vi "DAQmx-AI.GetPrivateEvents.vi"(8 "error in (no error)":errorcluster, 11 "DAQmx-AI":refnum<class "DAQmx-AI.lvclass">) -> (0 "error out":errorcluster, 2 "Private Events":T1, 3 "DAQmx-AI out":refnum<class "DAQmx-AI.lvclass">)   [LabVIEW 2016, in "DAQmx-AI.lvclass"]
doc: "---------------------------------------------------------------\nJKI State Machine Objects™\nhttp://jki.net/state-machine-objects/\nCopyright (C) 2005-2015, JKI <info@jki.net>\nALL RIGHTS RESERVEDJKI State Machine Objects (SMO) 1.0.0.5\nJKI - JKI\nCopyright (c) 2016, JKI"
uses:
  DAQmx-AI.lvclass
  Typedefs/PrivateEvents--Cluster.ctl
  Typedefs/Logging--Cluster.ctl
  DAQmx-AI.lvclass/DAQmx-AI.ctl
panel:
  # "For instructions on how to use the JKI State Machine Objects, examples and video tutorials, visit:\nhttp://jki.net/state-machine-objects/\n\nJKI State Machine Objects™\nhttp://jki.net/state-machine-objects/\nCopyright (C) 2005-2015, JKI <info@jki.net>\nALL RIGHTS RESERVED"
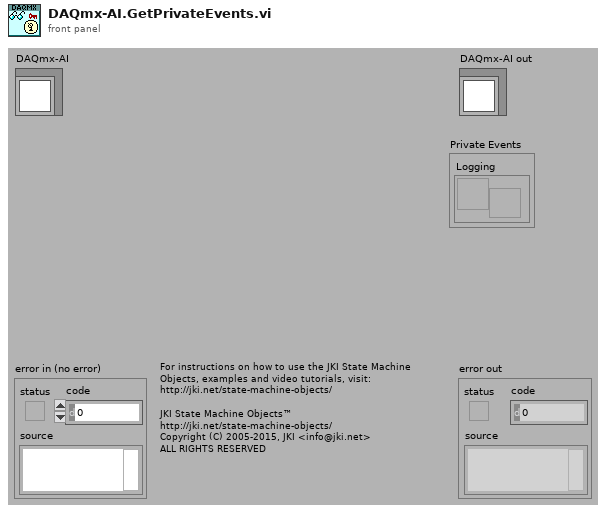
[diagram p1: front panel]
types:
  T1 = typedef "DAQmx-AI.lvclass/PrivateEvents--Cluster.ctl" = cluster{"Logging":refnum<user-event>}
  T2 = typedef "DAQmx-AI.lvclass/PrivateData--Ref.ctl" = refnum<data-value>
  T3 = typedef "DAQmx-AI.lvclass/PrivateData--Cluster.ctl" = cluster{"Configuration":T4, "Public Events":T6, "Data":dbl, "Scaling":T7, "Private Events":T1}
  T4 = typedef "DAQmx-AI.lvclass/Configuration--Cluster.ctl" = cluster{"PhysChan":tag, "Period (ms)":i64, "input terminal cfg":i32, "minimum value":dbl, "maximum value":dbl, "units":T5, "task name":string, "TDMS File Path":path, "Group Name":string}
  T5 = typedef "DAQmx-AI.lvclass/Units -- Enum.ctl" = enum16{"Volts", "Amps", "Deg F", "Deg C", "Deg R", "Kelvins", "Strain", "Ohms", "Hz", "Seconds", "Meters", "Inches", "Degrees", "Radians", "Ticks", "g", "m/s^2", "m/s", "in/s", "Pascals", "Newtons", "Pounds", "kgf", "psi", "bar", "Nm", "oz-in", "lb-in", "lb-ft", "Volts/Volt", "mVolts/Volt", "From TEDS"}
  T6 = typedef "DAQmx-AI.lvclass/PublicEvents--Cluster.ctl" = cluster{"Value Changed":refnum<user-event>, "Task Configuration":refnum<user-event>, "Scaling":refnum<user-event>}
  T7 = typedef "DAQmx-AI.lvclass/Scaling--Cluster.ctl" = cluster{"Scale Name":string, "Scale Type":T8, "Scaled Units":string, "Linear":T9, "Map Range":T10, "Polynomial":T11, "Table":T12}
  T8 = typedef "DAQmx-AI.lvclass/ScalingType--Enum.ctl" = enum16{"No scaling", "Linear", "Map Range", "Polynomial", "Table"}
  T9 = typedef "DAQmx-AI.lvclass/Scaling(Linear)--Cluster.ctl" = cluster{"Slope":dbl, "Intercept":dbl}
  T10 = typedef "DAQmx-AI.lvclass/Scaling(MapRange)--Cluster.ctl" = cluster{"Minimum":dbl, "Maximum":dbl}
  T11 = typedef "DAQmx-AI.lvclass/Scaling(Polynomial)--Cluster.ctl" = cluster{"forward coeff":dbl[], "reverse coeff":dbl[]}
  T12 = typedef "DAQmx-AI.lvclass/Scaling(Table)--Cluster.ctl" = cluster{"scaled values":dbl[], "pres-scaled values":dbl[]}
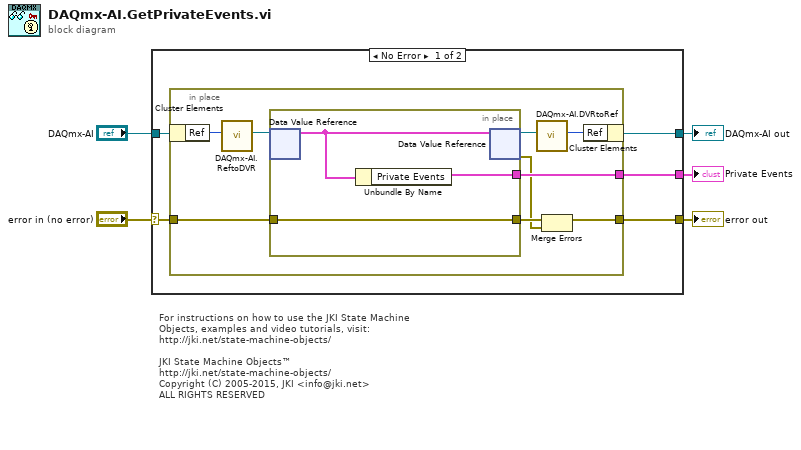
[diagram p0: block diagram]
diagram:
  # "For instructions on how to use the JKI State Machine Objects, examples and video tutorials, visit:\nhttp://jki.net/state-machine-objects/\n\nJKI State Machine Objects™\nhttp://jki.net/state-machine-objects/\nCopyright (C) 2005-2015, JKI <info@jki.net>\nALL RIGHTS RESERVED"
  n1 = case shown="No Error" "error in (no error)" {
    selector: "error in (no error)" -> [w9 w23]
    tunnel: "DAQmx-AI" -> [w10 w24]
    tunnel: [w6 w23] -> w4
    tunnel: [w8 w24] -> w3
    tunnel: [w7 _] -> w1
    frame No Error {
      n2 = in-place {
        in-place-border: w9 -> [w19]
        in-place-border: [w17] -> w6
        in-place-border: [w16] -> w7
        n3 = in-place-cluster #1(w10) -> ("Ref"=w14:u32)
        n4 = call "DAQmx-AI.ReftoDVR.vi"("Ref"=w14) -> ("Ref"=w13:T2)  [unwired: 10 in]
        n5 = in-place {
          in-place-border: w19 -> [w22]
          in-place-border: [w22] -> w18
          in-place-border: [w20] -> w16
          n6 = in-place-dvr #2(w13) -> (w21:T3)  [unwired: 1 out]
          n7 = Unbundle By Name(w21) -> ("Private Events"=w20:T1)
          n8 = in-place-dvr #2(w21) -> (w12:T2, w15:errorcluster)
        }
        n9 = call "DAQmx-AI.DVRtoRef.vi"("Ref"=w12) -> ("Ref"=w11:u32)  [unwired: 10 in]
        n10 = Merge Errors(w18, w15) -> (w17:errorcluster)
        n11 = in-place-cluster #1("Ref"=w11) -> (w8:refnum<class "DAQmx-AI.lvclass">)
      }
    }
    frame Error {
    }
  }
  "error out" <- w4
  "DAQmx-AI out" <- w3
  "Private Events" <- w1
